vi "GetPICoreTemperature.vi"(8 "error in (no error)":errorcluster) -> (0 "error out":errorcluster, 3 "PICoreTemp":dbl)   [LabVIEW 2014]
panel:
  out "standard error":string
  out "standard output":string
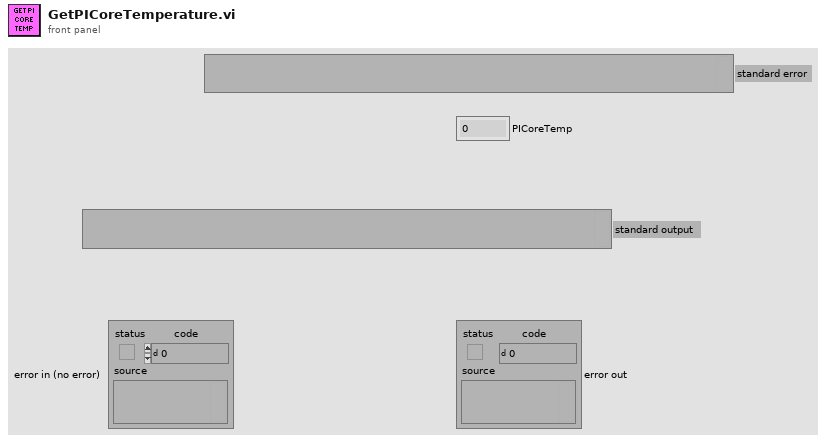
[diagram p1: front panel]
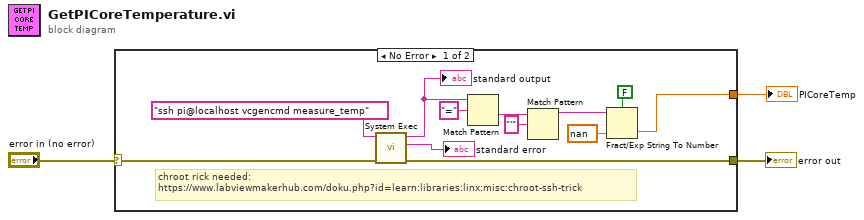
[diagram p0: block diagram]
diagram:
  n1 = case shown="No Error" "error in (no error)" {
    selector: "error in (no error)" -> [w14 w16]
    tunnel: [w15 w16] -> w3
    tunnel: [w7 _] -> w1
    frame No Error {
      # "chroot rick needed:\nhttps://www.labviewmakerhub.com/doku.php?id=learn:libraries:linx:misc:chroot-ssh-trick"
      n2 = call <vilib>:"System Exec.vi"("error in (no error)"=w14, "command line"="ssh pi@localhost vcgencmd measure_temp") -> ("error out"=w15:errorcluster, "standard error"=→"standard error":string, "standard output"=w13:string)  [unwired: 6 in, 1 out]
      "standard output" <- w13
      n3 = Match Pattern(string=w13, regular expression="=") -> (after substring=w11:string)  [unwired: 1 in, 3 out]
      n4 = Match Pattern(string=w11, regular expression="'") -> (before substring=w9:string)  [unwired: 1 in, 3 out]
      n5 = Fract/Exp String To Number(use system decimal point (T)=FALSE, string=w9, default (0 dbl)=nan ("default (0 DBL)")) -> (number=w7:dbl)  [unwired: 1 in, 1 out]
    }
    frame Error {
    }
  }
  "PICoreTemp" <- w1
  "error out" <- w3
